vi "Namen aus Tabelle ersetzen.vi"(8 "Fehler (Eingang, kein Fehler)":errorcluster, 9 "Regulärer Ausdruck":string, 10 "Sprachauswahl":u16, 11 "Tabelle":string[][](array[string])) -> (0 "Fehler (Ausgang)":errorcluster, 3 "Übersetzung":string)   [LabVIEW 2020, in "Sprachverwaltung.lvlib"]
uses:
  Sprachverwaltung.lvlib
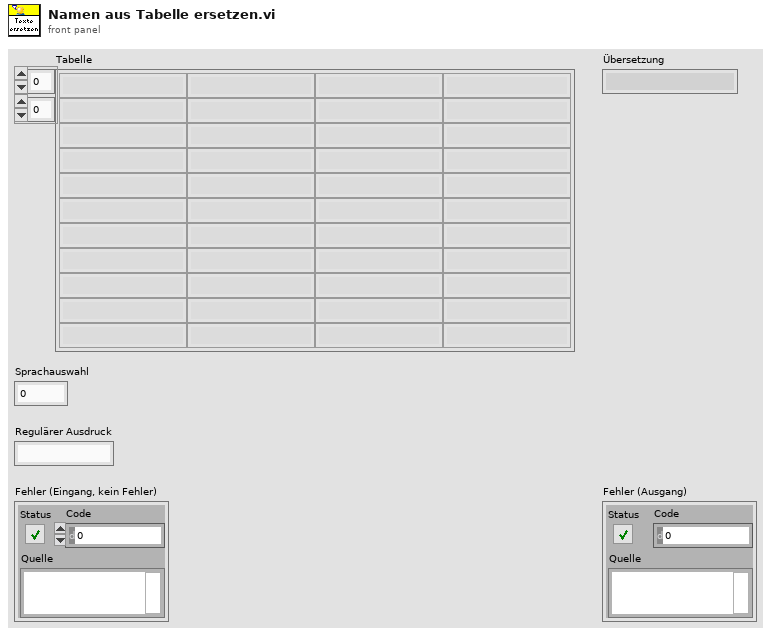
[diagram p1: front panel]
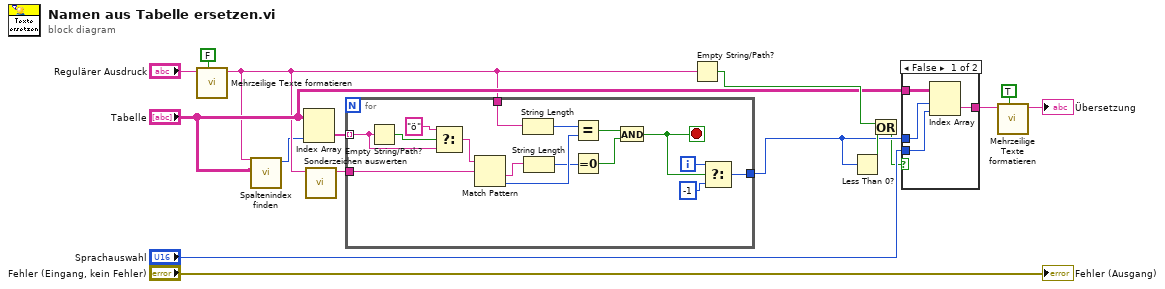
[diagram p0: block diagram]
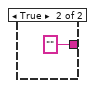
[diagram p2: hidden frame]
diagram:
  n1 = call "Mehrzeilige Texte formatieren.vi"("Zurück formatieren"=FALSE, "string"="Regulärer Ausdruck") -> ("result string"=w6:string)  [unwired: 9 in]
  n2 = call "Spaltenindex finden.vi"("Tabelle"="Tabelle", "Regulärer Ausdruck"=w6) -> ("Tab spalte"=w5:i32)  [unwired: 9 in]
  n3 = Index Array(array="Tabelle", index (col)=w5) -> (element=w14:string[])  [unwired: 1 in]
  n4 = call "Sonderzeichen auswerten.vi"("String"=w6) -> ("Suchstring"=w12:string)  [unwired: 9 in, 1 out]
  n5 = for {
    tunnel: w14 -> [w19] mode=indexing
    tunnel: w12 -> [w18]
    tunnel: w6 -> [w29]
    tunnel: [w25] -> w13
    i -> [w26]
    stop <- w24 stop-if-true
    n6 = Empty String/Path?(string/path=w19) -> (empty?=w32:bool)
    n7 = Select(t="ö", s=w32, f=w19) -> (s? t:f=w30:string)
    n8 = Match Pattern(string=w30, regular expression=w18) -> (after substring=w22:string, offset past match=w27:i32)  [unwired: 1 in, 2 out]
    n9 = String Length(string=w29) -> (length=w28:i32)
    n10 = String Length(string=w22) -> (length=w21:i32)
    n11 = Equal?(x=w28, y=w27) -> (x = y?=w23:bool)
    n12 = Equal To 0?(x=w21) -> (x = 0?=w20:bool)
    n13 = And(x=w23, y=w20) -> (x .and. y?=w24:bool)
    n14 = Select(t=w26, s=w24, f=-1) -> (s? t:f=w25:i32)
  }
  n15 = Empty String/Path?(string/path=w6) -> (empty?=w10:bool)
  n16 = Less Than 0?(x=w13) -> (x < 0?=w15:bool)
  n17 = Or(x=w10, y=w15) -> (x .or. y?=w11:bool)
  n18 = case shown="False" w11 {
    tunnel: [w36 "" ("String")] -> w3
    tunnel: "Sprachauswahl" -> [w35 _]
    tunnel: "Tabelle" -> [w34 _]
    tunnel: w13 -> [w33 _]
    frame False {
      n19 = Index Array(array=w34, index (row)=w33, index (col)=w35) -> (element=w36:string)
    }
    frame True {
    }
  }
  n20 = call "Mehrzeilige Texte formatieren.vi"("Zurück formatieren"=TRUE, "string"=w3) -> ("result string"=→"Übersetzung":string)  [unwired: 9 in]
  "Fehler (Ausgang)" <- "Fehler (Eingang, kein Fehler)"
